vi "GUI_HTU_Control_Center.vi"() -> ()   [LabVIEW 2013]
uses:
  shared programs/GUI_Template/GUI_master/tcp_new_data_event.ctl
  shared programs/GUI_Template/GUI_master/tcp new data cluster.ctl
  GUI_TestStand/Fire button.ctl
panel:
  out "Delay.Ch B::10":dbl caption="Opening time (s)" min=-0.1 max=0.1 format="%#_6p"
  in  "Set opening time (s)":dbl
  in  "Jet enable":bool caption="Jet Enable"
  in  "Position.Axis 3::6":dbl caption="Probe delay" min=0.0 max=25.0
  in  "Position.Axis 2::6":dbl caption="Jet Blade" min=-14.5 max=0.0
  in  "Position.Axis1::11":dbl caption="Compressor separation" min=-60000.0 max=60000.0
  in  "GUIdevice 11":string="U_CompAerotech"
  in  "pos.Channel1::9":enum16{"1", "2", "3", "4", "5", "6"}(ring) caption="Grating Mode filter"
  in  "pos.Channel3::5":enum16{"1", "2", "3", "4", "5", "6"}(ring) caption="Phasics"
  in  "pos.Channel2::5":enum16{"1", "2", "3", "4", "5", "6"}(ring) caption="Ghost pulsed"
  in  "pos.Channel1::5":enum16{"1", "2", "3", "4", "5", "6"}(ring) caption="Hamma Spec"
  in  "AnalogOutput.Channel 1::8":dbl caption="Pressure Control Voltage (V)" min=0.0 max=3.0
  in  "Position.Axis 3::7":dbl caption="Jet_Z" min=0.0 max=25.0
  in  "Position.Axis 2::7":dbl caption="Jet_Y" min=-25.0 max=0.0
  in  "Position.Axis 1::7":dbl caption="Jet_X" min=0.0 max=25.0
  in  "pos.Channel0::5":enum16{"1", "2", "3", "4", "5", "6"}(ring) caption="Mode Imager Filter"
  in  "Position.Channel 2::2":T1(ring) caption="Beamline In"
  in  "Position.Channel 1::2":T1(ring) caption="Beamline Out"
  in  "Position.Channel 6::1":T1(ring) caption="Gaia Beamblock 3-North"
  in  "Position.Channel 5::1":T1(ring) caption="Gaia Beamblock 4-North"
  in  "Position.Channel 4::1":T1(ring) caption="Gaia Stop South"
  in  "Position.Channel 3::1":T1(ring) caption="Gaia Stop North"
  in  "Position.Channel 2::1":T1(ring) caption="Gaia Beamblock 3-South"
  in  "Position.Channel 1::1":T1(ring) caption="Gaia Beamblock 4-South"
  in  "Position.Axis 1::6":dbl caption="Mode Imager Position" min=-60.0 max=20.0
  in  "Position.Axis 6::4":dbl caption="Beamline In Y" min=0.0 max=6.0
  in  "Position.Axis 5::4":dbl caption="Beamline In X" min=0.0 max=6.0
  in  "Position.Axis 4::4":dbl caption="Beamline Out Y" min=0.0 max=6.0
  in  "Position.Axis 3::4":dbl caption="Beamline Out X" min=0.0 max=6.0
  in  "Position.Axis 2::4":dbl caption="OAP In 2 Y" min=0.0 max=6.0
  in  "Position.Axis 1::4":dbl caption="OAP In 2 X" min=0.0 max=6.0
  in  "Position.Axis 6::3":dbl caption="OAP In 1 Y" min=0.0 max=6.0
  in  "Position.Axis 5::3":dbl caption="OAP In 1 X" min=0.0 max=6.0
  in  "Position.Axis 4::3":dbl caption="Comp In Y" min=0.0 max=6.0
  in  "Position.Axis 3::3":dbl caption="Comp In X" min=0.0 max=6.0
  in  "Position.Axis 2::3":dbl caption="Tube In Y" min=0.0 max=6.0
  in  "Position.Axis 1::3":dbl caption="Tube In X" min=0.0 max=6.0
  in  "GUIdevice 8":string="U_HP_Daq"
  in  "GUIdevice 6":string="U_ModeImagerESP"
  in  "GUIdevice 5":string="U_FilterWheel_01"
  in  "Fire Button":T2=TRUE
  out "error IO 2":errorcluster
  out "Amplitude.Ch AB::10":dbl caption="Amplitude Jet trigger" min=0.5 max=5.0 format="%.1f"
  out "fire::10":string
  out "tcp data event":T3
  in  "UDP error message":string
  in  "GUIdevice 7":string="U_ESP_JetXYZ"
  in  "GUIdevice 2":string="U_1Wire_Bcave"
  in  "GUIdevice 10":string="U_DG645_ShotControl"
  in  "GUIdevice 4":string="U_TRAServer02"
  in  "GUIdevice 1":string="U_1Wire_148"
  in  "GUIdevice 3":string="U_TRAServer01"
  in  "Step size":dbl min=-22.0 max=22.0 format="%.5f"
  in  "wangle::1":dbl caption="w (F11 F12)" min=-6.0 max=6.0 step=0.01 format="%.5f"
  in  "vangle::1":dbl caption="v (F9 F10)" min=-6.0 max=6.0 step=0.01 format="%.5f"
  in  "uangle::1":dbl caption="u (F7 F8)" min=-6.0 max=6.0 step=0.01 format="%.5f"
  in  "ypos::1":dbl caption="y (F3 F4)" min=-22.0 max=22.0 step=0.01 format="%.5f"
  in  "zpos::1":dbl caption="z (PgU PgD)" min=-12.0 max=12.0 step=0.01 format="%.5f"
  in  "xpos::1":dbl caption="x (F1 F2)" min=-22.0 max=22.0 step=0.01 format="%.5f"
  in  "Jet trigger":bool caption="Jet Trigger"
  in  "GUIdevice 9":string="U_FilterwheelGratingMode"
  in  "Delay.Ch C::10":dbl caption="Jet timing (s)" min=-0.1 max=0.1 format="%#_6p"
  in  "stop":bool
  # "HTU CONTROL CENTER"
  # "GAIA Flippers"
  # "B-Cave Alignement"
  # "Energy"
  # "Jet Stages"
  # "CAP"
  # "Mode Imager"
  # "\"-x\" is laser propagation direction"
  # "148 TRA motors"
  # "Jet timing and\n      trigger"
  # "Compressor"
  # "Filter Wheels"
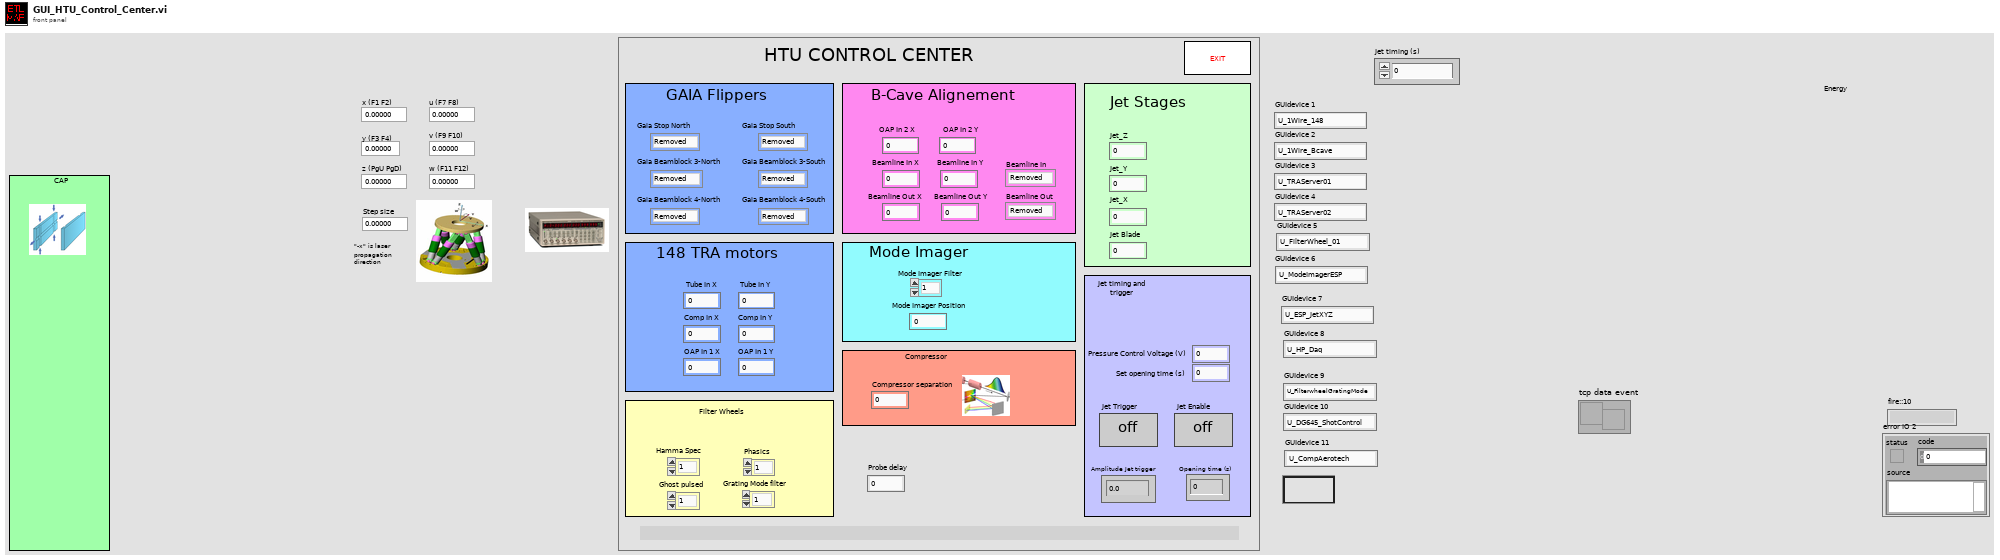
[diagram p1: front panel]
types:
  T1 = enum16{"Removed", "Inserted", "Unknown", "Moving"}
  T2 = typedef "Fire button.ctl" = bool
  T3 = typedef "tcp_new_data_event.ctl" = refnum<user-event>
  T4 = typedef "tcp new data cluster.ctl" = cluster{"EventEnum":enum16{"new data", "connection status update"}, "Device name":string}
  T5 = enum32{"invalid app kind", "Development System", "Run Time System", "Student Edition", "Embedded LabVIEW", "Evaluation", "Custom"}
  T6 = enum32{"Invalid", "Standard", "Closed", "Hidden", "Minimized", "Maximized"}
  T7 = cluster{"Core":cluster{"Current VI Reference":refnum<vi>, "Close Panel on Exit?":bool}, "Heater timing offset":dbl, "Discharge timing offset":dbl, "Jet trigger":bool, "Tik1":u32, "Tik2":u32, "Fire Continues Allowed":bool, "Jet enable":bool}
  T8 = cluster{"Current VI Reference":refnum<vi>, "Close Panel on Exit?":bool}
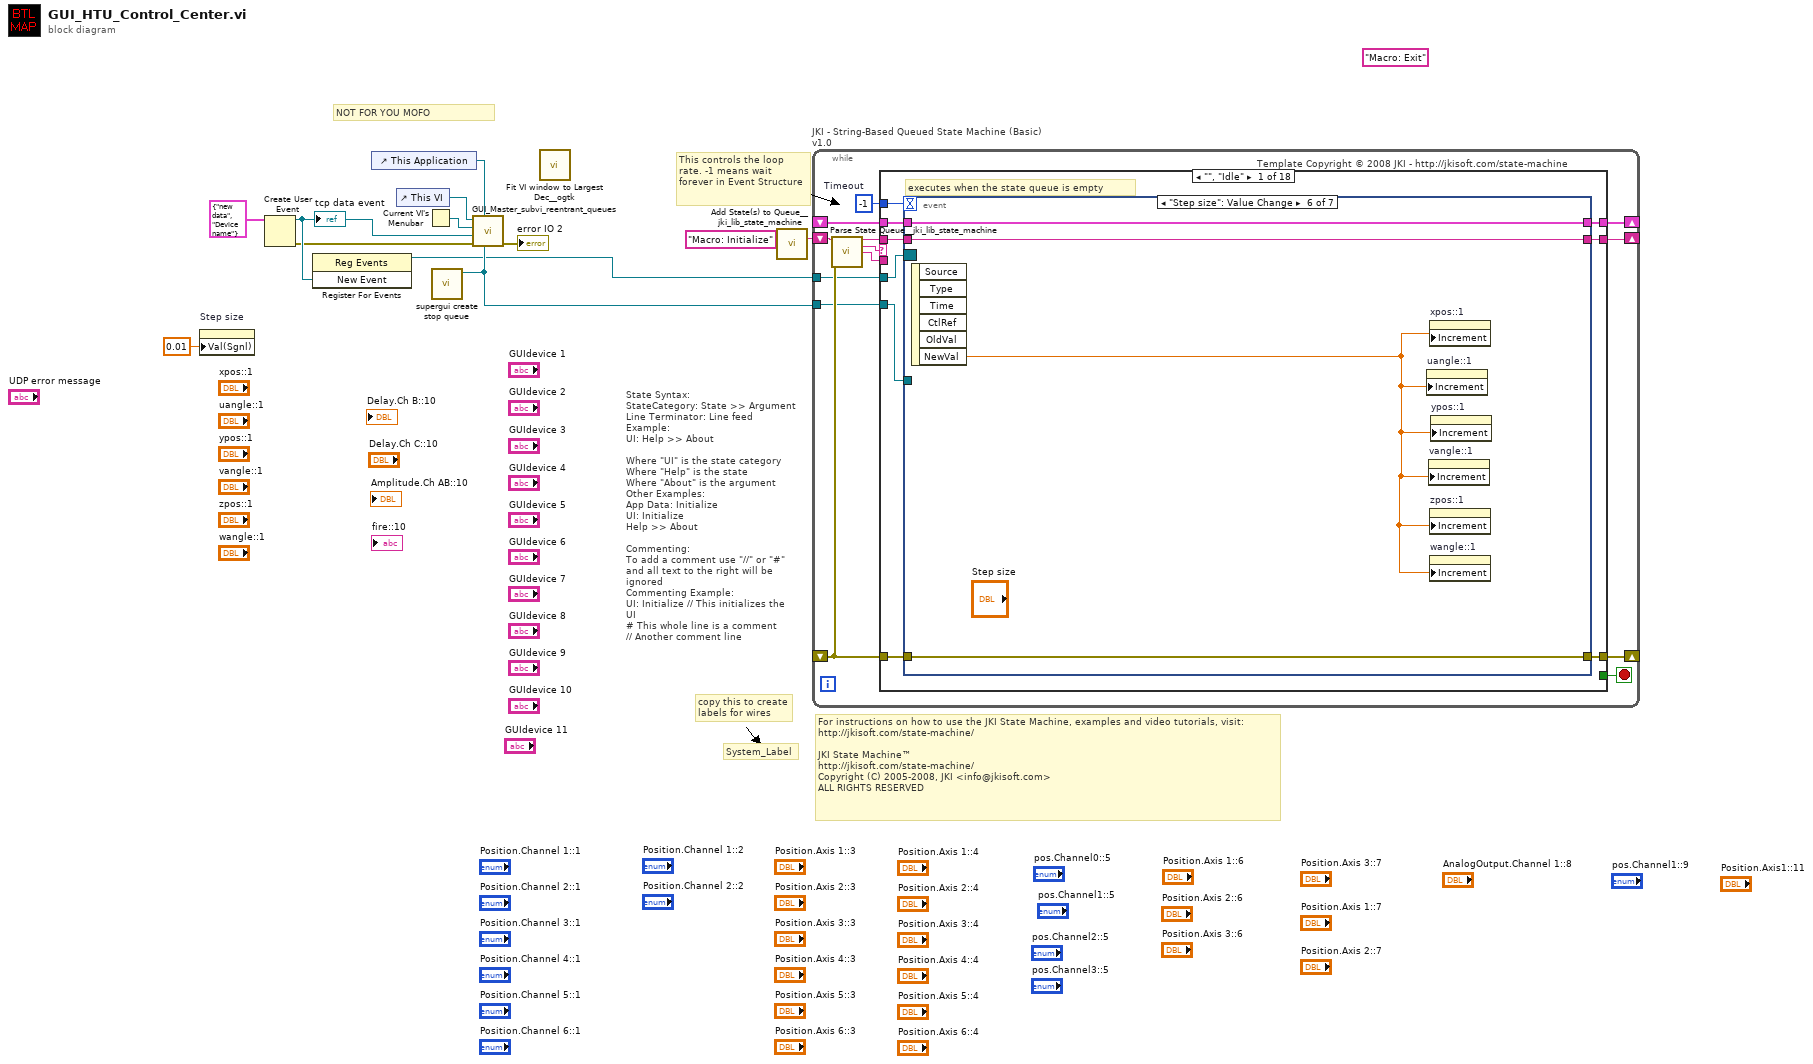
[diagram p0: block diagram]
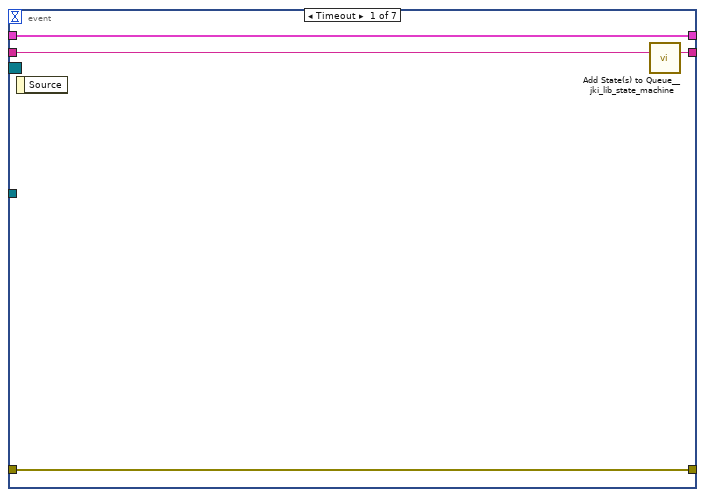
[diagram p2: hidden frame]
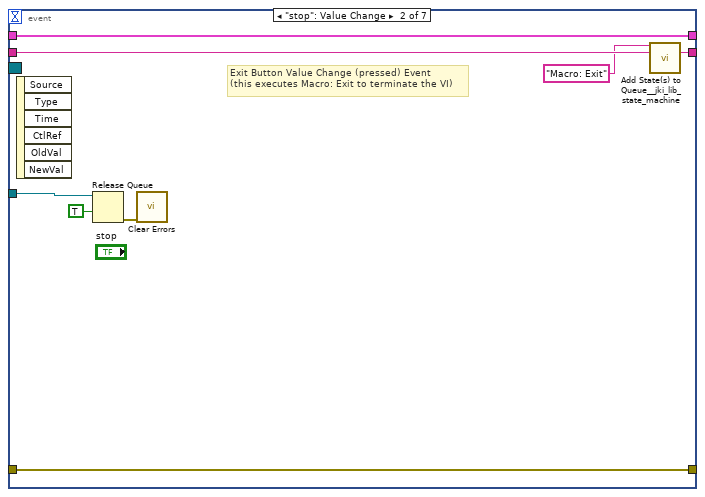
[diagram p3: hidden frame]
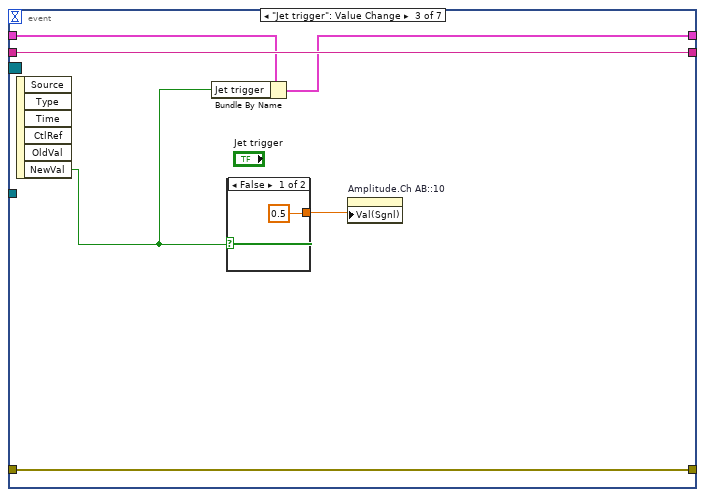
[diagram p4: hidden frame]
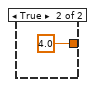
[diagram p5: hidden frame]
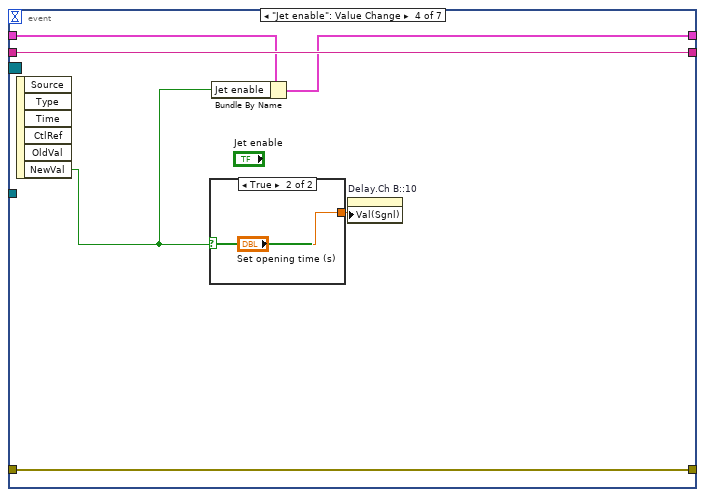
[diagram p6: hidden frame]
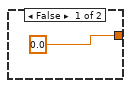
[diagram p7: hidden frame]
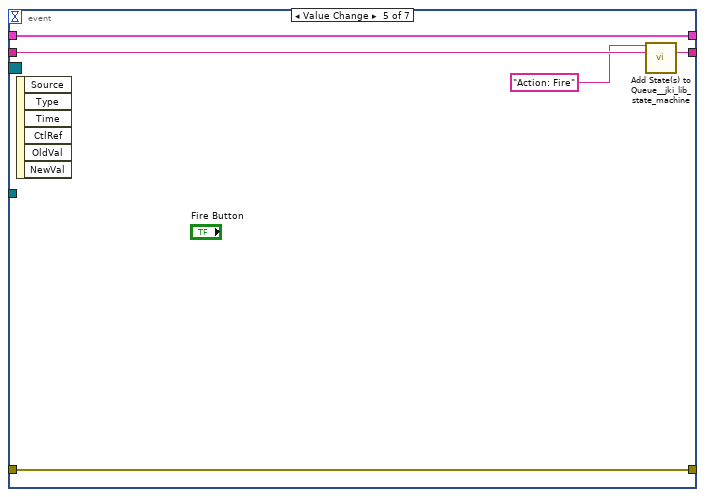
[diagram p8: hidden frame]
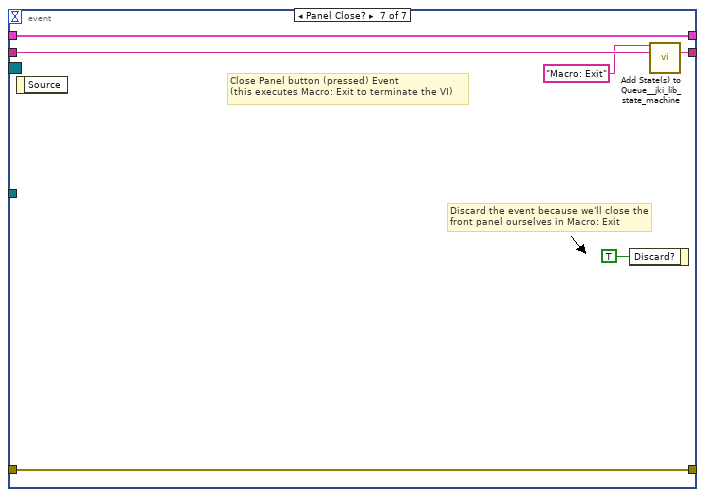
[diagram p9: hidden frame]
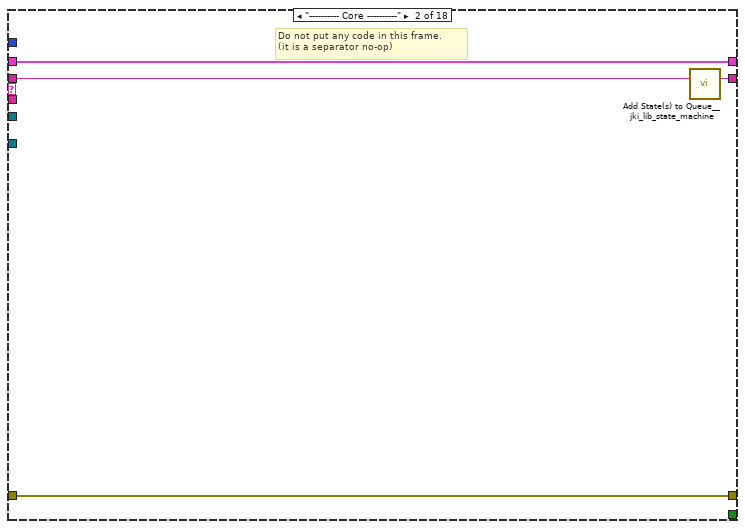
[diagram p10: hidden frame]
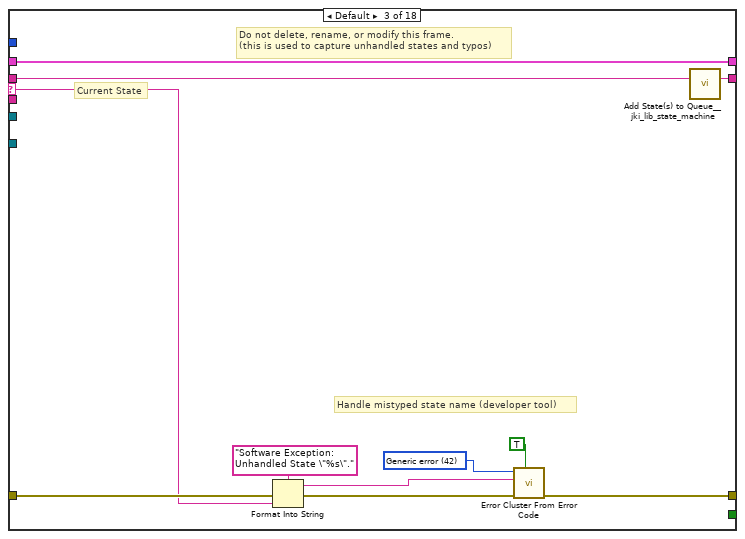
[diagram p11: hidden frame]
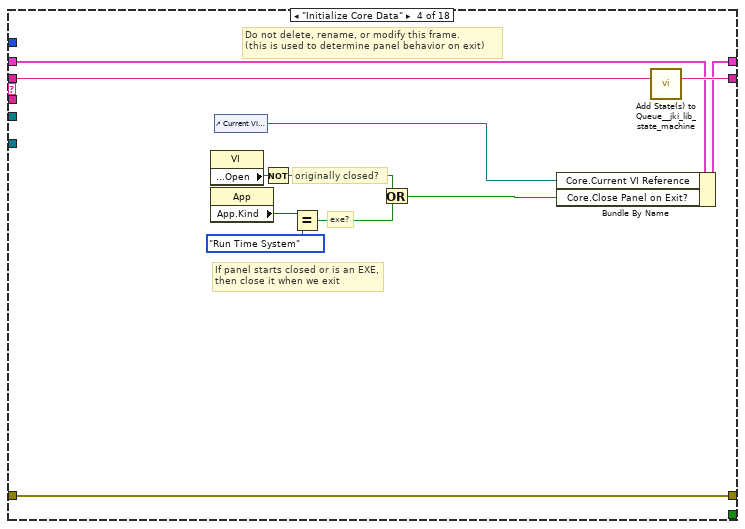
[diagram p12: hidden frame]
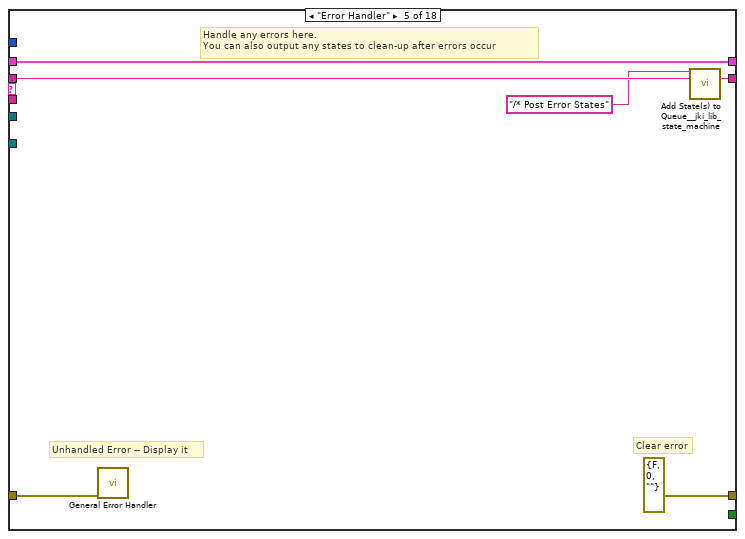
[diagram p13: hidden frame]
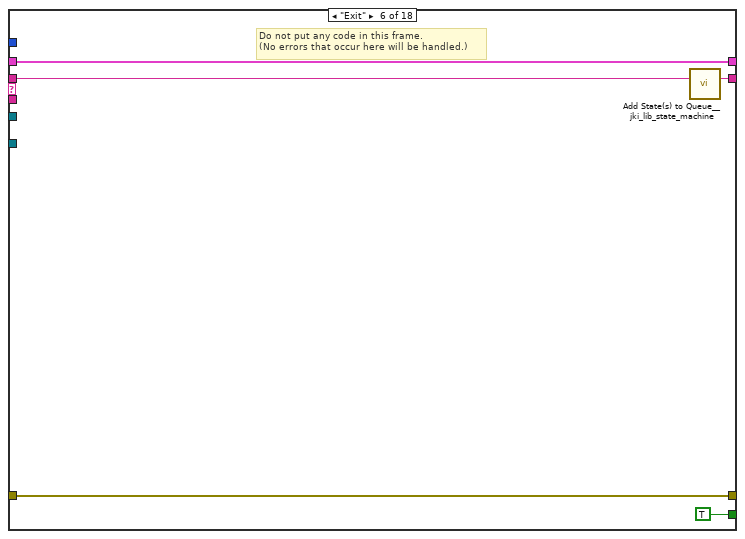
[diagram p14: hidden frame]
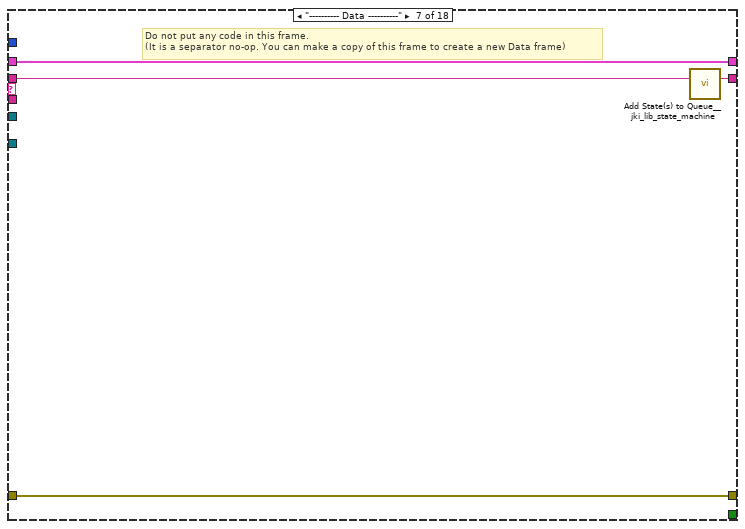
[diagram p15: hidden frame]
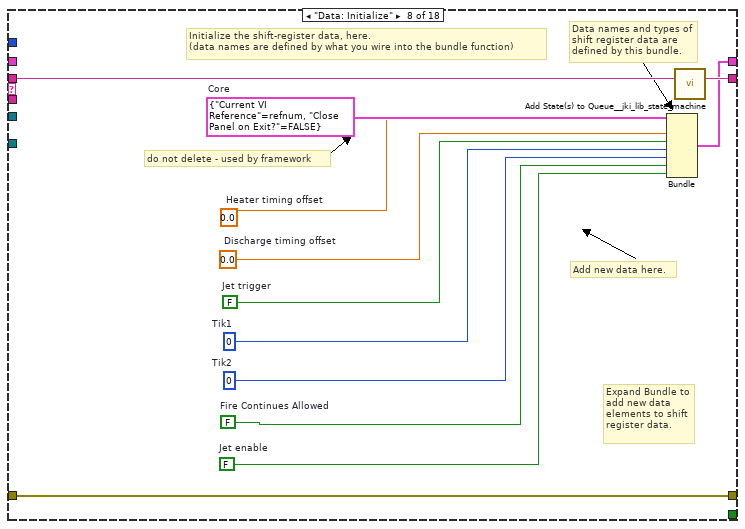
[diagram p16: hidden frame]
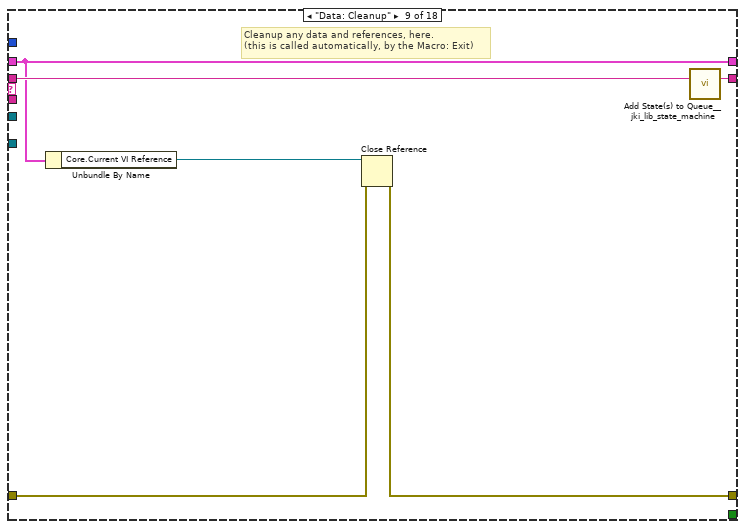
[diagram p17: hidden frame]
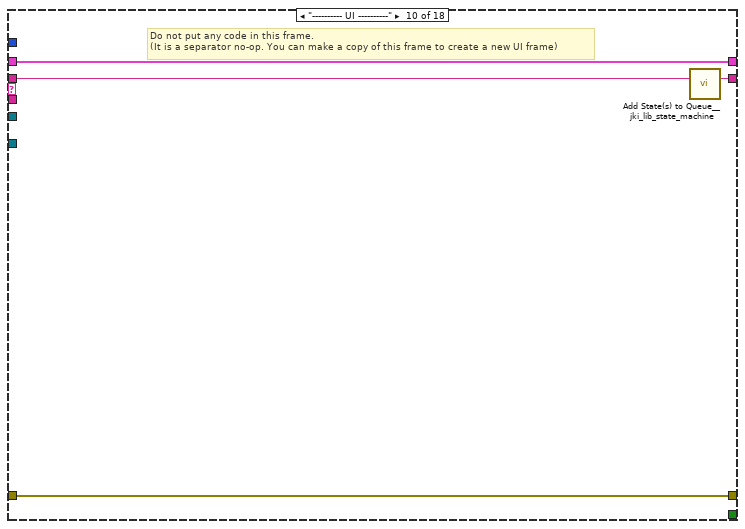
[diagram p18: hidden frame]
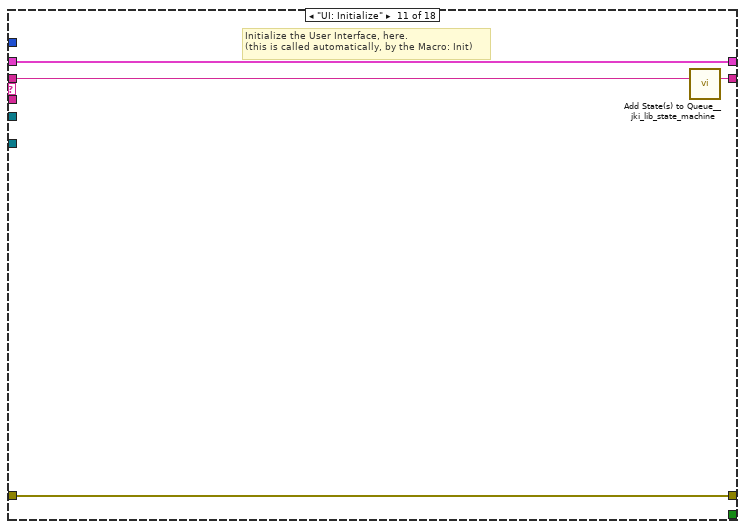
[diagram p19: hidden frame]
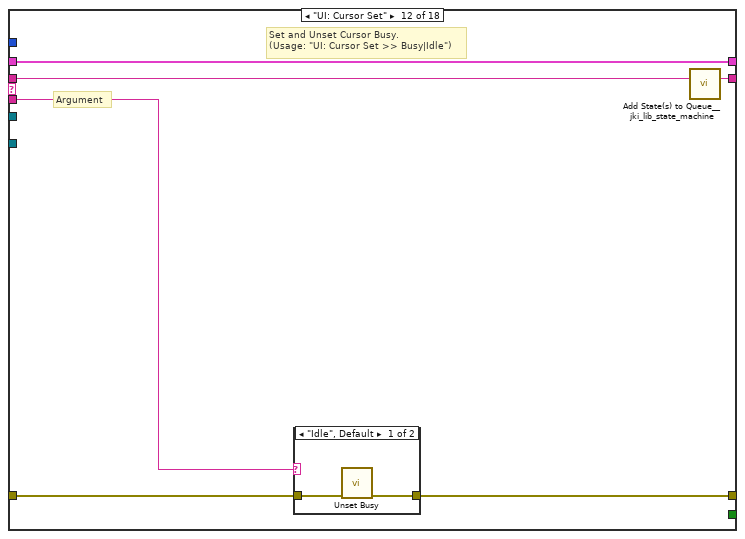
[diagram p20: hidden frame]
diagram:
  (unwired) "Macro: Exit"
  # "For instructions on how to use the JKI State Machine, examples and video tutorials, visit:\nhttp://jkisoft.com/state-machine/\n\nJKI State Machine™\nhttp://jkisoft.com/state-machine/\nCopyright (C) 2005-2008, JKI <info@jkisoft.com>\nALL RIGHTS RESERVED"
  # "State Syntax:\nStateCategory: State >> Argument\nLine Terminator: Line feed\nExample:\nUI: Help >> About\n\nWhere \"UI\" is the state category\nWhere \"Help\" is the state\nWhere \"About\" is the argument\nOther Examples:\nApp Data: Initialize\nUI: Initialize\nHelp >> About\n\nCommenting:\nTo add a comment use \"//\" or \"#\" and all text to the right will be ignored\nCommenting Example:\nUI: Initialize // This initializes the UI\n# This whole line is a comment\n// Another comment line"
  # "copy this to create labels for wires"
  # "This controls the loop rate. -1 means wait forever in Event Structure"
  # "System_Label"
  # "NOT FOR YOU MOFO"
  n1 = property on="Step size" class="DigNum (strict)"("Val(Sgnl)"=0.01 ("Value (Signaling)")) -> ()  [unwired: 2 in, 2 out]
  n2 = Create User Event(user event datatype=T4 {"EventEnum"=enum."new data", "Device name"="Device name"} ("New Event")) -> (user event=w11:refnum<user-event>, error out=w10:errorcluster)  [unwired: 1 in]
  "tcp data event" <- w11
  n3 = register-events(w11) -> (reference out=w1:refnum<event-registration>)  [unwired: 2 in, 1 out]
  n4 = control-ref of="This Application"() -> (w12:refnum<vi>)
  n5 = control-ref of="This VI"() -> (w5:refnum<vi>)
  n6 = Current VI's Menubar() -> (w8:refnum<k9>)
  n7 = call "supergui create stop queue.vi"() -> ("STOP Queue out"=w2:refnum<queue>)  [unwired: 11 in]
  n8 = call "GUI_Master_subvi_reentrant_queues.vi"("STOP Queue in"=w2, "This Application"=w12, "error in (no error)"=w10, "tcp data event"=w11, "Caller menu reference"=w8, "Caller VI ref"=w5) -> ("error out"=→"error IO 2":errorcluster)  [unwired: 5 in]
  n9 = call <userlib>:"Fit VI window to Largest Dec__ogtk.vi"() -> ()  [unwired: 6 in, 2 out]
  n10 = call <vilib>:"Add State(s) to Queue__jki_lib_state_machine.vi"("State(s) in (\"\")"="Macro: Initialize") -> ("States Out"=w3:string)  [unwired: 14 in]
  n11 = while "JKI - String-Based Queued State Machine (Basic) v1.0" {
    shift-right: [w18] -> _
    shift-left: _ -> [w17]
    shift-right: [w21] -> _
    shift-left: _ -> [w15]
    shift-right: [w20] -> _
    shift-left: w3 -> [w22]
    tunnel: w1 -> [w14]
    tunnel: w2 -> [w13]
    stop <- w19 stop-if-true
    w16 = -1  # Timeout
    # "Template Copyright © 2008 JKI - http://jkisoft.com/state-machine"
    n12 = call <vilib>:"Parse State Queue__jki_lib_state_machine.vi"("State Queue"=w22, "Error In (no error)"=w15) -> ("Remaining States"=w24:string, "Current State"=w25:string, "Arguments"=w23:string)  [unwired: 11 in]
    n13 = case shown="\"\", \"Idle\"" w25 {
      selector: w25 -> [_ _ w82 _ _ _ _ _ _ _ _ _ _ _ _ _ _ _]
      tunnel: w24 -> [w34 w81 w86 w104 w110 w115 w119 w131 w137 w141 w145 w151 w162 w188 w193 w203 w207 w213]
      tunnel: w23 -> [_ _ _ _ _ _ _ _ _ _ _ w146 w156 _ _ _ _ _]
      tunnel: w17 -> [w32 w78 w84 w95 w107 w113 w116 _ w132 w138 w143 w149 w158 w185 w190 w200 w204 w211]
      tunnel: [w31 w79 w88 w101 errorcluster {"status"=FALSE, "code"=0, "source"=""} ("error out") w112 w117 w128 w133 w139 w142 w147 w159 w186 w191 w201 w205 w208] -> w21
      tunnel: w15 -> [w30 w79 w87 w101 w106 w112 w117 w128 w134 w139 w142 w148 w160 w186 w191 w201 w205 w209]
      tunnel: [w33 w80 w85 w103 w109 w114 w118 w130 w136 w140 w144 w150 w161 w187 w192 w202 w206 w212] -> w20
      tunnel: [_ _ _ _ _ TRUE _ _ _ _ _ _ _ _ _ _ _ _] -> w19
      tunnel: [w26 w78 w84 w102 w107 w113 w116 w129 w132 w138 w143 w149 w158 w185 w190 w200 w204 w211] -> w18
      tunnel: w16 -> [w29 _ _ _ _ _ _ _ _ _ _ _ _ _ _ _ _ _]
      tunnel: w14 -> [w28 _ _ _ _ _ _ _ _ _ _ _ _ _ _ _ _ _]
      tunnel: w13 -> [w27 _ _ _ _ _ _ _ _ _ _ _ _ _ _ _ _ _]
      frame "", "Idle" {
        # "executes when the state queue is empty"
        n14 = event shown="[5] \"Step size\": Value Change" {
          selector: w28 -> [_ _ _ _ _ _ _]
          dyn-events: _ -> [_ _ _ _ _ _ _]
          timeout: w29 -> [_ _ _ _ _ _ _]
          tunnel: w34 -> [w38 w46 w52 w60 w64 w69 w77]
          tunnel: [w37 w45 w52 w60 w65 w69 w76] -> w33
          tunnel: w32 -> [w35 w43 w51 w59 w67 w70 w74]
          tunnel: [w36 w44 w47 w55 w66 w68 w75] -> w31
          tunnel: w30 -> [w36 w44 w47 w55 w66 w68 w75]
          tunnel: [w35 w43 w50 w58 w67 w70 w74] -> w26
          tunnel: w27 -> [_ w40 _ _ _ _ _]
          event Timeout {
            n15 = event-data() -> ()  [unwired: 1 in, 1 out]
            n16 = call <vilib>:"Add State(s) to Queue__jki_lib_state_machine.vi"("State(s) in (\"\")"=w38) -> ("States Out"=w37:string)  [unwired: 14 in]
          }
          event "stop": Value Change {
            # "Exit Button Value Change (pressed) Event\n(this executes Macro: Exit to terminate the VI)"
            n17 = event-data() -> ()  [unwired: 1 in, 6 out]
            n18 = Release Queue(queue=w40, force destroy? (F)=TRUE) -> (error out=w41:errorcluster)  [unwired: 1 in, 2 out]
            n19 = call <vilib>:"Clear Errors.vi"("error in (no error)"=w41) -> ()  [unwired: 6 in, 1 out]
            n20 = call <vilib>:"Add State(s) to Queue__jki_lib_state_machine.vi"("State(s) in Front (\"\")"="Macro: Exit", "State(s) in (\"\")"=w46) -> ("States Out"=w45:string)  [unwired: 13 in]
          }
          event "Jet trigger": Value Change {
            n21 = event-data() -> ("NewVal"=w49:bool)  [unwired: 1 in, 5 out]
            n22 = Bundle By Name(cluster=w51, "Jet trigger"=w49) -> (w50:T7)
            n23 = case shown="False" w49 {
              tunnel: [0.5 ("Amplitude.Ch CD::10") 4.0 ("Amplitude.Ch CD::10")] -> w48
              frame False {
              }
              frame True {
              }
            }
            n24 = property on="Amplitude.Ch AB::10" class="DigNum (strict)"("Val(Sgnl)"=w48) -> ()  [unwired: 2 in, 2 out]
          }
          event "Jet enable": Value Change {
            n25 = event-data() -> ("NewVal"=w57:bool)  [unwired: 1 in, 5 out]
            n26 = case shown="True" w57 {
              tunnel: [0.0 ("opening Time") "Set opening time (s)"] -> w56
              frame False {
              }
              frame True {
              }
            }
            n27 = Bundle By Name(cluster=w59, "Jet enable"=w57) -> (w58:T7)
            n28 = property on="Delay.Ch B::10" class="DigNum (strict)"("Val(Sgnl)"=w56) -> ()  [unwired: 2 in, 2 out]
          }
          event Value Change {
            n29 = event-data() -> ()  [unwired: 1 in, 6 out]
            n30 = call <vilib>:"Add State(s) to Queue__jki_lib_state_machine.vi"("State(s) in Front (\"\")"="Action: Fire" ("State(s) in Front (\"\")"), "State(s) in (\"\")"=w64) -> ("States Out"=w65:string)  [unwired: 13 in]
          }
          event "Step size": Value Change {
            n31 = event-data() -> ("NewVal"=w71:dbl)  [unwired: 1 in, 5 out]
            n32 = property on="uangle::1" class="DigNum (strict)"("Increment"=w71) -> ()  [unwired: 2 in, 2 out]
            n33 = property on="vangle::1" class="DigNum (strict)"("Increment"=w71) -> ()  [unwired: 2 in, 2 out]
            n34 = property on="xpos::1" class="DigNum (strict)"("Increment"=w71) -> ()  [unwired: 2 in, 2 out]
            n35 = property on="zpos::1" class="DigNum (strict)"("Increment"=w71) -> ()  [unwired: 2 in, 2 out]
            n36 = property on="wangle::1" class="DigNum (strict)"("Increment"=w71) -> ()  [unwired: 2 in, 2 out]
            n37 = property on="ypos::1" class="DigNum (strict)"("Increment"=w71) -> ()  [unwired: 2 in, 2 out]
          }
          event Panel Close? {
            # "Discard the event because we'll close the front panel ourselves in Macro: Exit"
            # "Close Panel button (pressed) Event\n(this executes Macro: Exit to terminate the VI)"
            n38 = event-data() -> ()  [unwired: 1 in, 1 out]
            n39 = event-data("Discard?"=TRUE) -> ()  [unwired: 1 in, 1 out]
            n40 = call <vilib>:"Add State(s) to Queue__jki_lib_state_machine.vi"("State(s) in Front (\"\")"="Macro: Exit", "State(s) in (\"\")"=w77) -> ("States Out"=w76:string)  [unwired: 13 in]
          }
        }
      }
      frame "---------- Core ----------" {
        # "Do not put any code in this frame.\n(it is a separator no-op)"
        n41 = call <vilib>:"Add State(s) to Queue__jki_lib_state_machine.vi"("State(s) in (\"\")"=w81) -> ("States Out"=w80:string)  [unwired: 14 in]
      }
      frame Default {
        w91 = 42 items=["No error", "Argument error", "Memory is full", "Out of zone", "End of file", "File already open", "Generic file I/O error", "File not found", "File permission error", "Disk is full", "Duplicate path", "Too many files open", "System feature not enabled", "Resource file not found", "Cannot add resource", "Resource not found", "Image not found", "Image memory error", "Pen does not exist", "Config type invalid", "Config token not found", "Config parse error", "Config memory error", "Bad external code format", "Bad external code offset", "External code not present", "Null window", "Destroy window error", "Null menu", "Print aborted", "Bad print record", "Print driver error", "Windows error during printing", "Memory error during printing", "Print dialog error", "Generic print error", "Invalid device refnum", "Device not found", "Device parameter error", "Device unit error", "Cannot open device", "Device call aborted", "Generic error", "Cancelled by user", "Object ID too low", "Object ID too high", "Object not in heap", "Unknown heap", "Unknown object (invalid DefProc)", "Unknown object (DefProc not in table)", "Message out of range", "Invalid (null) method", "Unknown message", "Manager call not supported", "Bad address", "Network operation in progress", "Network operation timed out", "Connection is busy", "Network attribute not supported", "Network error", "Address in use", "System out of memory", "Connection aborted", "Connection refused", "Not connected", "Already connected", "Connection closed", "Initialization error (interapplication manager)", "Bad occurrence", "Wait on unbound occurrence handler", "Occurrence queue overflow", "Datalog type conflict", "Unused", "Unrecognized type (interapplication manager)", "Memory corrupt", "Failed to make temporary DLL", "Old CIN version", "Drag socket not found", "Failed to load drop-object", "Failed to register OLE object", "Failed to release OLE object", "Format specifier type mismatch", "Unknown format specifier", "Too few format specifiers", "Too many format specifiers", "Scan failed", "Newer CIN version", "Error converting to variant", "Runtime menu error", "Password tampered", "Variant attribute not found", "Incompatible variant data type", "Event data is not available", "Event Store is not present", "Occurrence is not found", "Event Queue is not created", "Event info is not available", "Refnum passed is NULL", "Error retrieving Class GUID", "Error retrieving CoClass GUID", "Error retrieving TypeLib GUID.", "Bad built application magic bytes.", "Specific driver is different from the specific driver associated with the Logical Name.", "There is no session opened to the class driver.", "Max Error", "MAX - Error with config objects", "MAX - Error loading configuration", "MAX - Group not supported"]
        # "Current State"
        # "Do not delete, rename, or modify this frame.\n(this is used to capture unhandled states and typos)"
        # "Handle mistyped state name (developer tool)"
        n42 = Format Into String(format string="Software Exception: Unhandled State \"%s\"." ("message"), error in=w87, w82) -> (resulting string=w90:string, error out=w89:errorcluster)  [unwired: 1 in]
        n43 = call <vilib>:"Error Cluster From Error Code.vi"("show call chain? (False)"=TRUE, "error in (no error)"=w89, "error message (\"\")"=w90, "error code (0)"=w91) -> ("error out"=w88:errorcluster)  [unwired: 5 in]
        n44 = call <vilib>:"Add State(s) to Queue__jki_lib_state_machine.vi"("State(s) in (\"\")"=w86) -> ("States Out"=w85:string)  [unwired: 14 in]
      }
      frame "Initialize Core Data" {
        # "Do not delete, rename, or modify this frame.\n(this is used to determine panel behavior on exit)"
        # "originally closed?"
        # "exe?"
        # "If panel starts closed or is an EXE, then close it when we exit"
        n45 = property class="VI"() -> ("Front Panel.Open"=w100:bool)  [unwired: 2 in, 2 out]
        n46 = property class="App"() -> ("App.Kind"=w99:T5)  [unwired: 2 in, 2 out]
        n47 = control-ref of="Current VI Reference"() -> (w93:refnum<vi>)
        n48 = Not(x=w100) -> (.not. x?=w97:bool)
        n49 = Equal?(x=w99, y=T5."Run Time System" ("Application:Kind")) -> (x = y?=w96:bool)
        n50 = Or(x=w97, y=w96) -> (x .or. y?=w94:bool)
        n51 = Bundle By Name(cluster=w95, "Core.Current VI Reference"=w93, "Core.Close Panel on Exit?"=w94) -> (w102:T7)
        n52 = call <vilib>:"Add State(s) to Queue__jki_lib_state_machine.vi"("State(s) in (\"\")"=w104) -> ("States Out"=w103:string)  [unwired: 14 in]
      }
      frame "Error Handler" {
        # "Unhandled Error -- Display it"
        # "Handle any errors here.\nYou can also output any states to clean-up after errors occur"
        # "Clear error"
        n53 = call <vilib>:"General Error Handler.vi"("error in (no error)"=w106) -> ()  [unwired: 10 in, 5 out]
        n54 = call <vilib>:"Add State(s) to Queue__jki_lib_state_machine.vi"("State(s) in Front (\"\")"="/* Post Error States", "State(s) in (\"\")"=w110) -> ("States Out"=w109:string)  [unwired: 13 in]
      }
      frame "Exit" {
        # "Do not put any code in this frame.\n(No errors that occur here will be handled.)"
        n55 = call <vilib>:"Add State(s) to Queue__jki_lib_state_machine.vi"("State(s) in (\"\")"=w115) -> ("States Out"=w114:string)  [unwired: 14 in]
      }
      frame "---------- Data ----------" {
        # "Do not put any code in this frame.\n(It is a separator no-op. You can make a copy of this frame to create a new Data frame)"
        n56 = call <vilib>:"Add State(s) to Queue__jki_lib_state_machine.vi"("State(s) in (\"\")"=w119) -> ("States Out"=w118:string)  [unwired: 14 in]
      }
      frame "Data: Initialize" {
        w120 = FALSE  # Jet enable
        w121 = FALSE  # Fire Continues Allowed
        w123 = u32 0  # Tik1
        w122 = u32 0  # Tik2
        w124 = FALSE  # Jet trigger
        w125 = 0.0  # Discharge timing offset
        w126 = 0.0  # Heater timing offset
        w127 = T8 {"Current VI Reference"=refnum, "Close Panel on Exit?"=FALSE}  # Core
        # "do not delete - used by framework"
        # "Expand Bundle to add new data elements to shift register data."
        # "Add new data here."
        # "Data names and types of shift register data are defined by this bundle."
        # "Initialize the shift-register data, here.\n(data names are defined by what you wire into the bundle function)"
        n57 = Bundle("Core"=w127, "Heater timing offset"=w126, "Discharge timing offset"=w125, "Jet trigger"=w124, "Tik1"=w123, "Tik2"=w122, "Fire Continues Allowed"=w121, "Jet enable"=w120) -> (w129:T7)  [unwired: 1 in]
        n58 = call <vilib>:"Add State(s) to Queue__jki_lib_state_machine.vi"("State(s) in (\"\")"=w131) -> ("States Out"=w130:string)  [unwired: 14 in]
      }
      frame "Data: Cleanup" {
        # "Cleanup any data and references, here.\n(this is called automatically, by the Macro: Exit)"
        n59 = Unbundle By Name(w132) -> ("Core.Current VI Reference"=w135:refnum<vi>)
        n60 = Close Reference(reference=w135, error in (no error)=w134) -> (error out=w133:errorcluster)
        n61 = call <vilib>:"Add State(s) to Queue__jki_lib_state_machine.vi"("State(s) in (\"\")"=w137) -> ("States Out"=w136:string)  [unwired: 14 in]
      }
      frame "---------- UI ----------" {
        # "Do not put any code in this frame.\n(It is a separator no-op. You can make a copy of this frame to create a new UI frame)"
        n62 = call <vilib>:"Add State(s) to Queue__jki_lib_state_machine.vi"("State(s) in (\"\")"=w141) -> ("States Out"=w140:string)  [unwired: 14 in]
      }
      frame "UI: Initialize" {
        # "Initialize the User Interface, here.\n(this is called automatically, by the Macro: Init)"
        n63 = call <vilib>:"Add State(s) to Queue__jki_lib_state_machine.vi"("State(s) in (\"\")"=w145) -> ("States Out"=w144:string)  [unwired: 14 in]
      }
      frame "UI: Cursor Set" {
        # "Argument"
        # "Set and Unset Cursor Busy.\n(Usage: \"UI: Cursor Set >> Busy|Idle\")"
        n64 = case shown="\"Idle\", Default" w146 {
          tunnel: w148 -> [w153 w155]
          tunnel: [w152 w154] -> w147
          frame "Idle", Default {
            n65 = call <vilib>:"Unset Busy.vi"("error in (no error)"=w153) -> ("error out"=w152:errorcluster)  [unwired: 10 in]
          }
          frame "Busy" {
            n66 = call <vilib>:"Set Busy.vi"("error in (no error)"=w155) -> ("error out"=w154:errorcluster)  [unwired: 9 in, 1 out]
          }
        }
        n67 = call <vilib>:"Add State(s) to Queue__jki_lib_state_machine.vi"("State(s) in (\"\")"=w151) -> ("States Out"=w150:string)  [unwired: 14 in]
      }
      frame "UI: Front Panel State" {
        # "Argument"
        # "Set Front Panel Open or Closed\n(Usage: \"UI: Front Panel State >> Open|Close\")"
        n68 = Unbundle By Name(w158) -> ("Core.Current VI Reference"=w157:refnum<vi>)
        n69 = case shown="\"Close\"" w156 {
          tunnel: w160 -> [w166 w179]
          tunnel: [w168 w180] -> w159
          tunnel: w157 -> [w167 w177]
          frame "Open", Default {
            n70 = property class="VI"(reference=w167, error in=w166) -> (reference out=w164:refnum<vi>, error out=w165:errorcluster, "Front Panel.Open"=w163:bool)
            n71 = case shown="False" w163 {
              tunnel: [w171 w174] -> w168
              tunnel: w165 -> [w170 w174]
              tunnel: w164 -> [w169 _]
              frame False {
                n72 = invoke class="VI" method="FP.Open"(reference=w169, error in=w170, "Activate"=TRUE, "State"=T6."Standard") -> (error out=w171:errorcluster)  [unwired: 1 in, 4 out]
              }
              frame True {
              }
            }
          }
          frame "Close" {
            n73 = property class="VI"(reference=w177, error in=w179) -> (reference out=w176:refnum<vi>, error out=w178:errorcluster, "Front Panel.Open"=w175:bool)
            n74 = case shown="True" w175 {
              tunnel: [w181 w184] -> w180
              tunnel: w178 -> [w181 w183]
              tunnel: w176 -> [_ w182]
              frame False {
              }
              frame True {
                n75 = invoke class="VI" method="FP.Close"(reference=w182, error in=w183) -> (error out=w184:errorcluster)  [unwired: 1 in, 2 out]
              }
            }
          }
        }
        n76 = call <vilib>:"Add State(s) to Queue__jki_lib_state_machine.vi"("State(s) in (\"\")"=w162) -> ("States Out"=w161:string)  [unwired: 14 in]
      }
      frame "---------- Macro ----------" {
        # "Do not put any code in this frame.\n(It is a separator no-op. You can make a copy of this frame to create a new Macro frame)"
        n77 = call <vilib>:"Add State(s) to Queue__jki_lib_state_machine.vi"("State(s) in (\"\")"=w188) -> ("States Out"=w187:string)  [unwired: 14 in]
      }
      frame "Macro: Initialize" {
        w189 = "Data: Initialize\nInitialize Core Data\nUI: Initialize\nUI: Front Panel State >> Open"  # Data: Initialize Initialize Core Data UI: Initialize UI: Front Panel State >> Open
        # "Initialization Macro\n(This is called once, when the VI starts)"
        n78 = call <vilib>:"Add State(s) to Queue__jki_lib_state_machine.vi"("State(s) in Front (\"\")"=w189, "State(s) in (\"\")"=w193) -> ("States Out"=w192:string)  [unwired: 13 in]
      }
      frame "Macro: Exit" {
        # "Exit Macro\n(This is called once, when the VI exits)"
        n79 = Unbundle By Name(w200) -> ("Core.Close Panel on Exit?"=w199:bool)
        n80 = Select(t="UI: Front Panel State >> Close", s=w199, f="") -> (s? t:f=w196:string)
        n81 = call <vilib>:"Add State(s) to Queue__jki_lib_state_machine.vi"("State(s) in (\"\")"=w196, "State(s) at Back (\"\")"="Data: Cleanup\nExit") -> ("States Out"=w194:string)  [unwired: 13 in]
        n82 = call <vilib>:"Add State(s) to Queue__jki_lib_state_machine.vi"("State(s) in Front (\"\")"=w194, "State(s) in (\"\")"=w203) -> ("States Out"=w202:string)  [unwired: 13 in]
      }
      frame "---------- New Category ----------" {
        # "Template Separator\n(You can make a copy of, or modify, this frame)"
        n83 = call <vilib>:"Add State(s) to Queue__jki_lib_state_machine.vi"("State(s) in (\"\")"=w207) -> ("States Out"=w206:string)  [unwired: 14 in]
      }
      frame "Action: Fire" {
        # "Your code here.\n(You can make a copy of, or modify, this frame)"
        n84 = property on="fire::10" class="Str"(error in=w209, "Val(Sgnl)"="fire>>force" ("Value (Signaling)")) -> (error out=w208:errorcluster)  [unwired: 1 in, 1 out]
        n85 = call <vilib>:"Add State(s) to Queue__jki_lib_state_machine.vi"("State(s) in (\"\")"=w213) -> ("States Out"=w212:string)  [unwired: 14 in]
      }
    }
  }
